vi "Power Set Request.vi"(8 "error in (no error)":errorcluster, 10 "Power Request Type":T1, 11 "Handle in":i64) -> (0 "error out":errorcluster, 2 "Success?":bool, 3 "Handle out":i64)   [LabVIEW 2024, in "Request Power.lvlib"]
uses:
  Request Power.lvlib
  typedefs/Power Request Type.ctl
  kernel32.dll
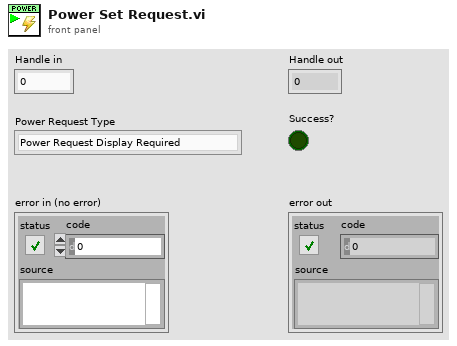
[diagram p1: front panel]
types:
  T1 = typedef "Request Power.lvlib/Power Request Type.ctl" = enum32{"Power Request Display Required", "Power Request System Required", "Power Request Away Mode Required", "Power Request Execution Required"}
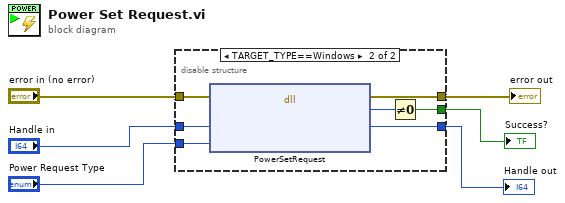
[diagram p0: block diagram]
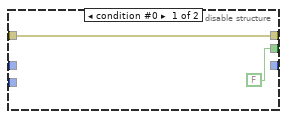
[diagram p2: hidden frame]
diagram:
  n1 = disable-structure shown="TARGET_TYPE==Windows" {
    disable-tunnel: [w8 w15] -> w6
    disable-tunnel: "error in (no error)" -> [w8 w14]
    disable-tunnel: "Handle in" -> [_ w13]
    disable-tunnel: "Power Request Type" -> [_ w12]
    disable-tunnel: [FALSE w10] -> w2
    disable-tunnel: [_ w9] -> w1
    frame condition #0 {
    }
    frame condition #1 (active) {
      n2 = dll-call lib="kernel32.dll" fn="PowerSetRequest"(error in=w14, "_In_ HANDLE"=w13, "_In_ POWER_REQUEST_TYPE"=w12) -> (error out=w15:errorcluster, "BOOL"=w11:i32, "_In_ HANDLE"=w9:i64)  [unwired: 3 in, 1 out]
      n3 = Not Equal To 0?(x=w11) -> (x != 0?=w10:bool)
    }
  }
  "error out" <- w6
  "Success?" <- w2
  "Handle out" <- w1
